vi "MDF_Set_Default_Install.vi"(8 "error in (no error)":errorcluster, 11 "userFolder in":refnum<class "userFolder.lvclass">) -> (0 "error out":errorcluster)   [LabVIEW 2020, in "userFolder.lvclass"]
uses:
  <vilib>/AppBuilder/IB_Classes/Destination/userFolder/userFolder.lvclass
  <vilib>/AppBuilder/IB_Classes/Destination/userFolder/userFolder.lvclass/userFolder.ctl
  <vilib>/AppBuilder/IB_Classes/Destination/IB_Destination.lvclass
  AppLibs/distkit/MDF/NIMdf.llb/MDFBDPAddFilePathType.ctl
  AppLibs/distkit/MDF/NI_MDF.lvlib
  AppLibs/distkit/MDF/NIMdf.llb/MDFBuildDevPart_SetDefaultInstallDir (string).vi
  e:/builds/penguin/labview/branches/2020/dev/dist/vi.lib/AppBuilder/IB_Classes/Destination/IB_Destination.lvclass
  e:/builds/penguin/labview/branches/2020/dev/dist/vi.lib/AppBuilder/IB_Classes/Destination/userFolder/userFolder.lvclass
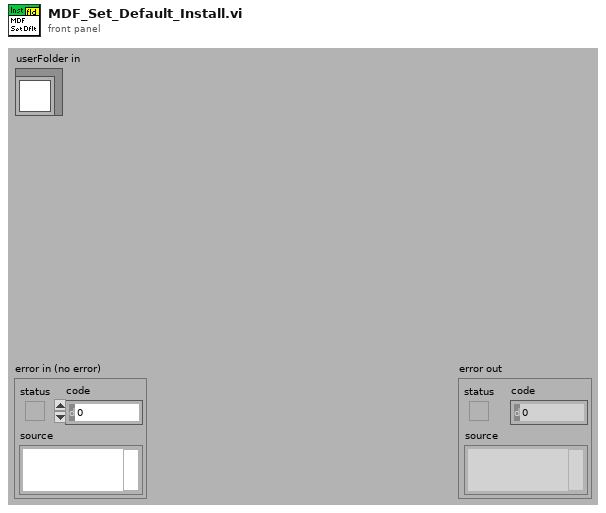
[diagram p1: front panel]
types:
  T1 = typedef "IB_Destination.ctl" = cluster{"name":string, "unlock":bool, "parentTag":string, "destTag":string, "eng_installPath":string}
  T2 = typedef "NI_MDF.lvlib/MDFBDPAddFilePathType.ctl" = i32
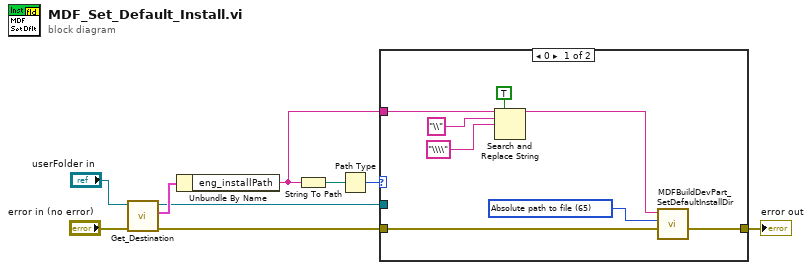
[diagram p0: block diagram]
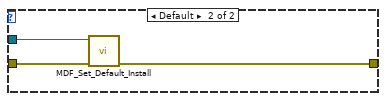
[diagram p2: hidden frame]
diagram:
  n1 = call <vilib>:"Get_Destination.vi"("error in (no error)"="error in (no error)", "IB_Destination in"="userFolder in") -> ("error out"=w4:errorcluster, "data"=w7:T1, "IB_Destination out"=w2:refnum<class "userFolder.lvclass">)  [unwired: 7 in]
  n2 = Unbundle By Name(w7) -> ("eng_installPath"=w1:string)
  n3 = String To Path(string=w1) -> (path=w9:path)
  n4 = Path Type(1:w9) -> (0:w8:i16)
  n5 = case shown="0" w8 {
    tunnel: w4 -> [w16 w19]
    tunnel: [w16 w18] -> w3
    tunnel: w2 -> [_ w17]
    tunnel: w1 -> [w13 _]
    frame 0 {
      w15 = T2 65 items=["Relative to default installation directory"=68, "Root directory on first partition"=70, "Relative to directory table key"=82, "Absolute path to file"=65] ("installation directory path type (Root directory on first partition)")
      n6 = Search and Replace String(replace all?=TRUE ("replace all? (F)"), input string=w13, search string="\\", replace string="\\\\" ("replace string (\"\")")) -> (result string=w14:string)  [unwired: 4 in, 3 out]
      n7 = call-poly "MDFBuildDevPart_SetDefaultInstallDir.vi"("installation directory path type (Root directory on first partition)"=w15, "default installation directory"=w14) -> ()  [unwired: 9 in, 1 out]
    }
    frame Default {
      n8 = call-parent "MDF_Set_Default_Install.vi"("error in (no error)"=w19, "IB_Destination in"=w17) -> ("error out"=w18:errorcluster)  [unwired: 9 in]
    }
  }
  "error out" <- w3
